vi "Send Command.vi"(8 "Error In":errorcluster, 9 "ARGS":u8[](array[numeric]), 10 "CMD":u16, 11 "LINX Device Config":T1) -> (0 "Error Out":errorcluster, 2 "Packet":u8[](array[numeric]), 3 "LINX Device Config":T1)   [LabVIEW 2011, in "LVH-LINX.lvlib"]
doc: "Send a packet to the LINX device and return the LINX device response packet."
uses:
  LVH-LINX.lvlib
  Type Defs/LINX Device Config.ctl
  Type Defs/Interface.ctl
  Type Defs/TCP Config.ctl
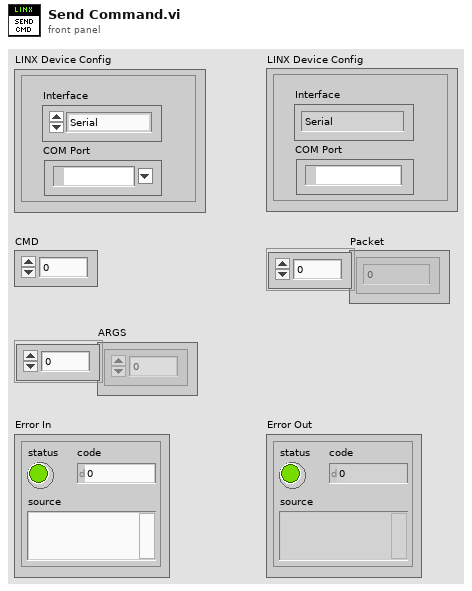
[diagram p1: front panel]
types:
  T1 = typedef "LVH-LINX.lvlib/LINX Device Config.ctl" = cluster{"Interface":T2, "COM Port":refnum<visa-resource-name>, "Packet Number":u16, "TCP Configuration":T3}
  T2 = typedef "LVH-LINX.lvlib/Interface.ctl" = enum16{"Serial", "TCP"}
  T3 = typedef "LVH-LINX.lvlib/TCP Config.ctl" = cluster{"IP Address":string, "Port":dbl}
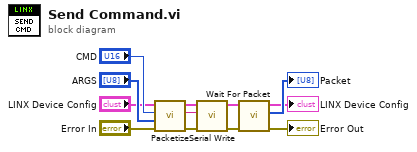
[diagram p0: block diagram]
diagram:
  n1 = call "Packetize.vi"("Error In"="Error In", "ARGS"="ARGS", "CMD"="CMD", "LINX Device Config"="LINX Device Config") -> ("Error Out"=w11:errorcluster, "Packet"=w8:string, "LINX Decice Config"=w12:T1)  [unwired: 5 in]
  n2 = call "Serial Write.vi"("Error In"=w11, "Data"=w8, "LINX Device Config"=w12) -> ("Error Out"=w10:errorcluster, "LINX Device Config"=w9:T1)  [unwired: 7 in]
  n3 = call "Wait For Packet.vi"("Error In"=w10, "LINX Device Config"=w9) -> ("Error Out"=→"Error Out":errorcluster, "Packet"=→"Packet":u8[], "LINX Device Config"=→"LINX Device Config":T1)  [unwired: 7 in]
